vi "Convert to Binary Display.vi"(6 "Variant in":variant, 7 "Shift Pressed?":bool, 8 "error in (no error)":errorcluster, 10 "QD Combo Box Ref":refnum<vi>, 11 "QD Launch VI Ref":refnum<vi>) -> (0 "error out":errorcluster, 4 "Variant out":variant)   [LabVIEW 2017, in "Control Operation.lvlib"]
doc: "Changes the display format of the selected string and numeric controls and indicators to binary."
uses:
  Control Operation.lvlib
panel:
  in  "Undo Name":string="Quick Drop Keyboard Shortcut"
  # "Do not change the connector pane of this VI.\n\nSee the block diagram for directions on how to use this template."
  # "Specify the name of the Undo transaction"
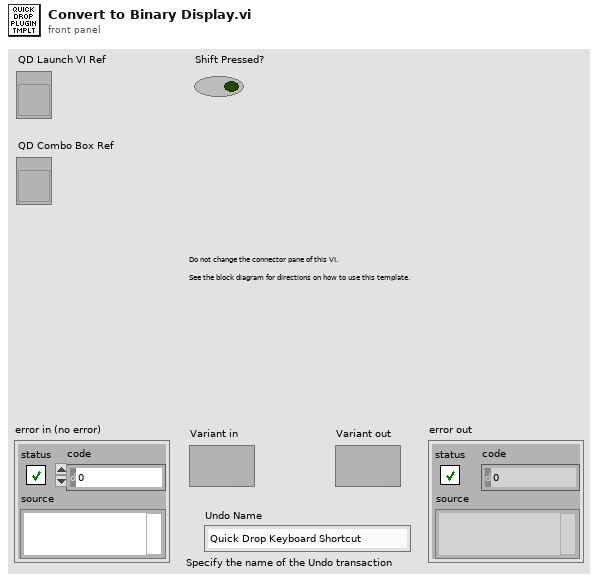
[diagram p1: front panel]
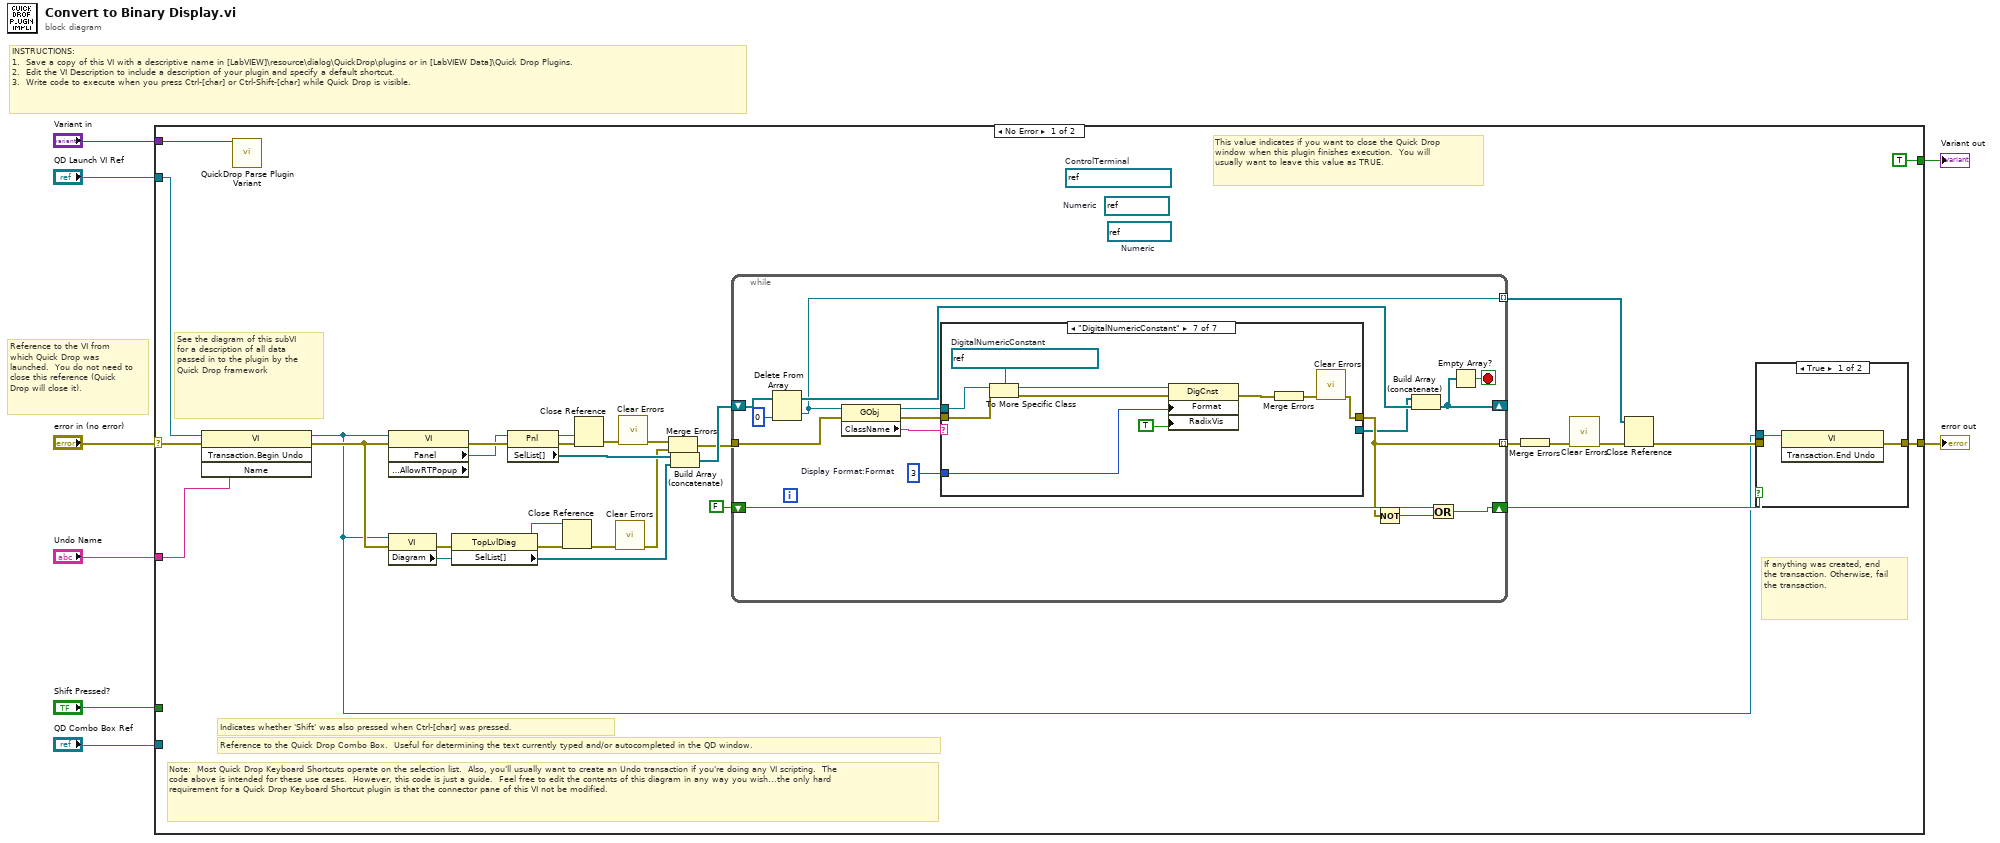
[diagram p0: block diagram]
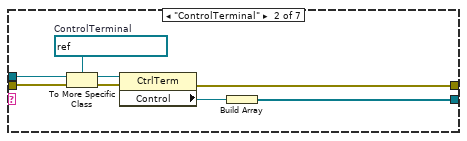
[diagram p3: hidden frame]
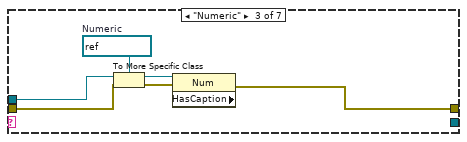
[diagram p4: hidden frame]
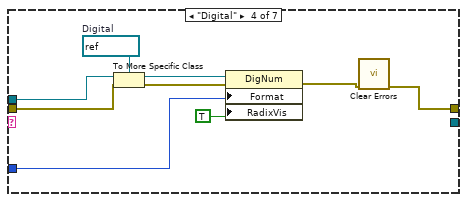
[diagram p5: hidden frame]
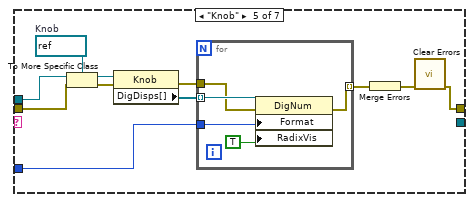
[diagram p6: hidden frame]
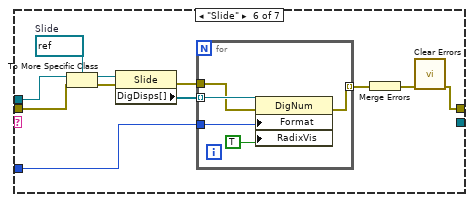
[diagram p7: hidden frame]
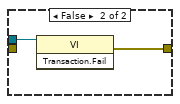
[diagram p8: hidden frame]
diagram:
  # "Reference to the VI from which Quick Drop was launched.  You do not need to close this reference (Quick Drop will close it)."
  # "INSTRUCTIONS:\n1.  Save a copy of this VI with a descriptive name in [LabVIEW]\\resource\\dialog\\QuickDrop\\plugins or in [LabVIEW Data]\\Quick Drop Plugins.\n2.  Edit the VI Description to include a description of your plugin and specify a default shortcut. \n3.  Write code to execute when you press Ctrl-[char] or Ctrl-Shift-[char] while Quick Drop is visible."
  n1 = case shown="No Error" "error in (no error)" {
    selector: "error in (no error)" -> [w38 w126]
    tunnel: [w34 w126] -> w7
    tunnel: "QD Launch VI Ref" -> [w37 _]
    tunnel: "Shift Pressed?" -> [_ _]
    tunnel: "QD Combo Box Ref" -> [_ _]
    tunnel: "Variant in" -> [w39 _]
    tunnel: "Undo Name" -> [w36 _]
    tunnel: [TRUE _] -> w1
    frame No Error {
      (unwired) refnum<vi> refnum  # Numeric
      (unwired) refnum<vi> refnum  # Numeric
      (unwired) refnum<vi> refnum  # ControlTerminal
      # "Note:  Most Quick Drop Keyboard Shortcuts operate on the selection list.  Also, you'll usually want to create an Undo transaction if you're doing any VI scripting.  The code above is intended for these use cases.  However, this code is just a guide.  Feel free to edit the contents of this diagram in any way you wish...the only hard requirement for a Quick Drop Keyboard Shortcut plugin is that the connector pane of this VI not be modified."
      # "If anything was created, end the transaction. Otherwise, fail the transaction."
      # "This value indicates if you want to close the Quick Drop window when this plugin finishes execution.  You will usually want to leave this value as TRUE."
      # "See the diagram of this subVI for a description of all data passed in to the plugin by the Quick Drop framework"
      # "Reference to the Quick Drop Combo Box.  Useful for determining the text currently typed and/or autocompleted in the QD window."
      # "Indicates whether 'Shift' was also pressed when Ctrl-[char] was pressed."
      n2 = invoke class="VI" method="Transaction.Begin Undo"(reference=w37, error in=w38, "Name"=w36) -> (reference out=w17:refnum<vi>, error out=w18:errorcluster)  [unwired: 1 in, 2 out]
      n3 = call <vilib>:"QuickDrop Parse Plugin Variant.vi"("QDKS Variant in"=w39) -> ()  [unwired: 12 in, 3 out]
      n4 = property class="VI" props=["Panel", "Front Panel.AllowRTPopup"](reference=w17, error in=w18) -> (error out=w30:errorcluster, "Panel"=w29:refnum<vi>)  [unwired: 2 out]
      n5 = property class="VI"(reference=w17, error in=w18) -> (error out=w22:errorcluster, "Diagram"=w21:refnum<vi>)  [unwired: 1 out]
      n6 = property class="TopLvlDiag"(reference=w21, error in=w22) -> (reference out=w19:refnum<vi>, error out=w20:errorcluster, "SelList[]"=w15:refnum<vi>[])
      n7 = property class="Pnl"(reference=w29, error in=w30) -> (reference out=w27:refnum<vi>, error out=w28:errorcluster, "SelList[]"=w25:refnum<vi>[])
      n8 = Close Reference(reference=w19, error in (no error)=w20) -> (error out=w10:errorcluster)
      n9 = Close Reference(reference=w27, error in (no error)=w28) -> (error out=w9:errorcluster)
      n10 = call <vilib>:"Clear Errors.vi"("error in (no error)"=w10) -> ("error out"=w12:errorcluster)  [unwired: 5 in, 1 out]
      n11 = call <vilib>:"Clear Errors.vi"("error in (no error)"=w9) -> ("error out"=w13:errorcluster)  [unwired: 5 in, 1 out]
      n12 = Merge Errors(w13, w12) -> (w14:errorcluster)
      n13 = Build Array (concatenate)(w25, w15) -> (w16:refnum<vi>[])
      n14 = while {
        shift-right: [w54] -> w32
        shift-left: FALSE -> [w55]
        tunnel: w14 -> [w51]
        tunnel: [w53] -> w26 mode=indexing
        shift-right: [w42] -> _
        shift-left: w16 -> [w47]
        tunnel: [w43] -> w11 mode=indexing
        stop <- w41 stop-if-true
        w40 = u8 3  # Display Format:Format
        n15 = Delete From Array(array=w47, index=0) -> (deleted portion=w43:refnum<vi>, array with subset deleted=w45:refnum<vi>[])  [unwired: 1 in]
        n16 = property class="GObj"(reference=w43, error in=w51) -> (reference out=w49:refnum<vi>, error out=w50:errorcluster, "ClassName"=w48:string)
        n17 = case shown="\"DigitalNumericConstant\"" w48 {
          tunnel: [w56 w57 w67 w73 w85 w101 w118] -> w53
          tunnel: w50 -> [w56 w61 w66 w75 w87 w103 w120]
          tunnel: w49 -> [_ w60 w65 w74 w86 w102 w119]
          tunnel: [_ w58 _ _ _ _ _] -> w44
          tunnel: w40 -> [_ _ _ w71 w80 w96 w112]
          frame Default {
          }
          frame "ControlTerminal" {
            w62 = refnum<vi> refnum  # ControlTerminal
            n18 = To More Specific Class(target class=w62, reference=w60, error in=w61) -> (specific class reference=w64:refnum<vi>, error out=w63:errorcluster)
            n19 = property class="CtrlTerm"(reference=w64, error in=w63) -> (error out=w57:errorcluster, "Control"=w59:refnum<vi>)  [unwired: 1 out]
            n20 = Build Array(w59) -> (w58:refnum<vi>[])
          }
          frame "Numeric" {
            w70 = refnum<vi> refnum  # Numeric
            n21 = To More Specific Class(target class=w70, reference=w65, error in=w66) -> (specific class reference=w69:refnum<vi>, error out=w68:errorcluster)
            n22 = property class="Num" props=["HasCaption"](reference=w69, error in=w68) -> (error out=w67:errorcluster)  [unwired: 2 out]
          }
          frame "Digital" {
            w79 = refnum<vi> refnum  # Digital
            n23 = To More Specific Class(target class=w79, reference=w74, error in=w75) -> (specific class reference=w78:refnum<vi>, error out=w77:errorcluster)
            n24 = property class="DigNum"(reference=w78, error in=w77, "Format"=w71, "RadixVis"=TRUE ("Radix Visible?")) -> (error out=w76:errorcluster)  [unwired: 1 out]
            n25 = call <vilib>:"Clear Errors.vi"("error in (no error)"=w76) -> ("error out"=w73:errorcluster)  [unwired: 5 in, 1 out]
          }
          frame "Knob" {
            w90 = refnum<vi> refnum  # Knob
            n26 = To More Specific Class(target class=w90, reference=w86, error in=w87) -> (specific class reference=w89:refnum<vi>, error out=w88:errorcluster)
            n27 = property class="Knob"(reference=w89, error in=w88) -> (error out=w83:errorcluster, "DigDisps[]"=w84:refnum<vi>[])  [unwired: 1 out]
            n28 = for {
              tunnel: w84 -> [w94] mode=indexing
              tunnel: w83 -> [w93]
              tunnel: [w92] -> w82 mode=indexing
              tunnel: w80 -> [w91]
              n29 = property class="DigNum"(reference=w94, error in=w93, "Format"=w91, "RadixVis"=TRUE ("Radix Visible?")) -> (error out=w92:errorcluster)  [unwired: 1 out]
            }
            n30 = Merge Errors(w82) -> (w81:errorcluster)
            n31 = call <vilib>:"Clear Errors.vi"("error in (no error)"=w81) -> ("error out"=w85:errorcluster)  [unwired: 5 in, 1 out]
          }
          frame "Slide" {
            w106 = refnum<vi> refnum  # Slide
            n32 = To More Specific Class(target class=w106, reference=w102, error in=w103) -> (specific class reference=w105:refnum<vi>, error out=w104:errorcluster)
            n33 = property class="Slide"(reference=w105, error in=w104) -> (error out=w99:errorcluster, "DigDisps[]"=w100:refnum<vi>[])  [unwired: 1 out]
            n34 = for {
              tunnel: w100 -> [w110] mode=indexing
              tunnel: w99 -> [w109]
              tunnel: [w108] -> w98 mode=indexing
              tunnel: w96 -> [w107]
              n35 = property class="DigNum"(reference=w110, error in=w109, "Format"=w107, "RadixVis"=TRUE ("Radix Visible?")) -> (error out=w108:errorcluster)  [unwired: 1 out]
            }
            n36 = Merge Errors(w98) -> (w97:errorcluster)
            n37 = call <vilib>:"Clear Errors.vi"("error in (no error)"=w97) -> ("error out"=w101:errorcluster)  [unwired: 5 in, 1 out]
          }
          frame "DigitalNumericConstant" {
            w121 = refnum<vi> refnum  # DigitalNumericConstant
            n38 = To More Specific Class(target class=w121, reference=w119, error in=w120) -> (specific class reference=w113:refnum<vi>, error out=w115:errorcluster)
            n39 = property class="DigCnst"(reference=w113, error in=w115, "Format"=w112, "RadixVis"=TRUE ("Radix Visible?")) -> (error out=w117:errorcluster)  [unwired: 1 out]
            n40 = Merge Errors(w117) -> (w116:errorcluster)
            n41 = call <vilib>:"Clear Errors.vi"("error in (no error)"=w116) -> ("error out"=w118:errorcluster)  [unwired: 5 in, 1 out]
          }
        }
        n42 = Not(x=w53) -> (.not. x?=w52:bool)
        n43 = Build Array (concatenate)(w44, w45) -> (w42:refnum<vi>[])
        n44 = Or(x=w55, y=w52) -> (x .or. y?=w54:bool)
        n45 = Empty Array?(array=w42) -> (empty?=w41:bool)
      }
      n46 = Merge Errors(w26) -> (w24:errorcluster)
      n47 = call <vilib>:"Clear Errors.vi"("error in (no error)"=w24) -> ("error out"=w23:errorcluster)  [unwired: 5 in, 1 out]
      n48 = Close Reference(reference=w11, error in (no error)=w23) -> (error out=w33:errorcluster)
      n49 = case shown="True" w32 {
        tunnel: w17 -> [w122 w124]
        tunnel: [w123 w125] -> w34
        tunnel: w33 -> [_ _]
        frame True {
          n50 = invoke class="VI" method="Transaction.End Undo"(reference=w122) -> (error out=w123:errorcluster)  [unwired: 2 in, 2 out]
        }
        frame False {
          n51 = invoke class="VI" method="Transaction.Fail"(reference=w124) -> (error out=w125:errorcluster)  [unwired: 2 in, 2 out]
        }
      }
    }
    frame Error {
    }
  }
  "error out" <- w7
  "Variant out" <- w1
